vi "Get GUI Control.vi"(8 "error in (no error)":errorcluster, 11 "Control Builder in":refnum<class "GUI Control Builder.lvclass">) -> (0 "error out":errorcluster, 2 "GUI Control":refnum<class "GUI Control.lvclass">, 3 "Control Builder out":refnum<class "GUI Control Builder.lvclass">)   [LabVIEW 2015, in "GUI Control Builder.lvclass"]
uses:
  GUI Control Builder.lvclass
  GUI Controls/GUI Control/GUI Control.lvclass
  GUI Control Builder.lvclass/GUI Control Builder.ctl
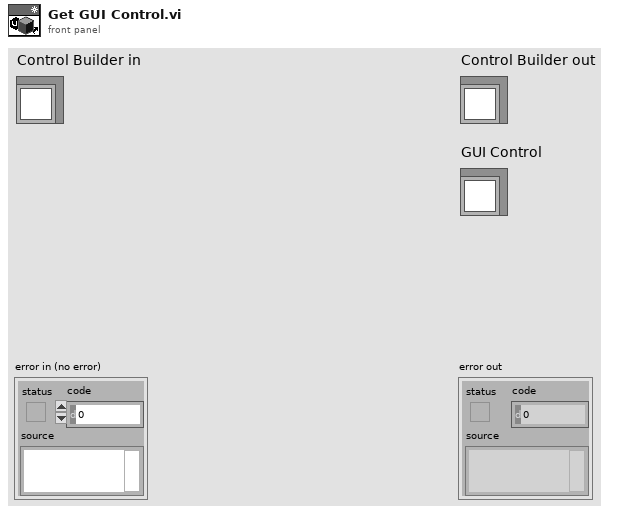
[diagram p1: front panel]
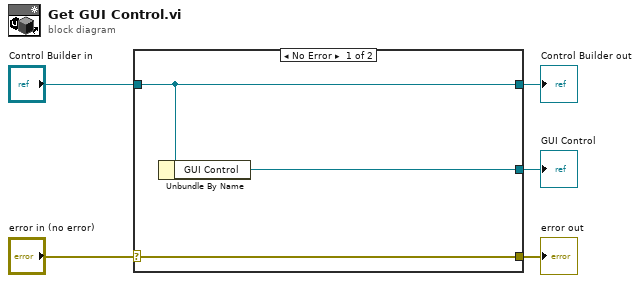
[diagram p0: block diagram]
diagram:
  n1 = case shown="No Error" "error in (no error)" {
    selector: "error in (no error)" -> [w8 w9]
    tunnel: [w8 w9] -> w4
    tunnel: [w7 w10] -> w2
    tunnel: "Control Builder in" -> [w7 w10]
    tunnel: [w6 _] -> w1
    frame No Error {
      n2 = Unbundle By Name(w7) -> ("GUI Control"=w6:refnum<class "GUI Control.lvclass">)
    }
    frame Error {
    }
  }
  "error out" <- w4
  "Control Builder out" <- w2
  "GUI Control" <- w1
